vi "get position calb.vi"(8 "error in (no error)":errorcluster, 9 "calibration":cluster{"A":dbl, "MicrostepMode":u32}, 10 "the_get_position_calb":T1, 11 "id":i32) -> (0 "error out":errorcluster, 2 "the_get_position_calb out":T1, 3 "function return":i32)   [LabVIEW 2012, in "libximc.lvlib"]
doc: "result_t XIMC_API get_position_calb (device_t id, get_position_calb_t* the_get_position_calb, const calibration_t* calibration);"
uses:
  libximc.lvlib
  libximc.dll
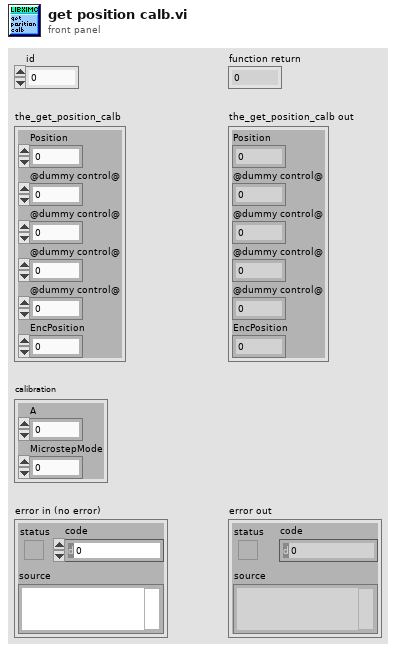
[diagram p1: front panel]
types:
  T1 = cluster{"Position":sgl, "@dummy control@":i8, "@dummy control@":i8, "@dummy control@":i8, "@dummy control@":i8, "EncPosition":i64}
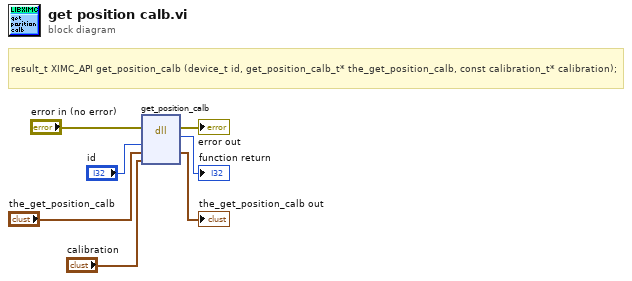
[diagram p0: block diagram]
diagram:
  # "result_t XIMC_API get_position_calb (device_t id, get_position_calb_t* the_get_position_calb, const calibration_t* calibration);"
  n1 = dll-call lib="C:/Users/user/Desktop/labview-2.9.11-gen/libximc.*" fn="get_position_calb"(error in="error in (no error)", "id"="id", "the_get_position_calb"="the_get_position_calb", "calibration"="calibration") -> (error out=→"error out":errorcluster, →"function return":i32, "the_get_position_calb"=→"the_get_position_calb out":T1)  [unwired: 4 in, 1 out]
